vi "DetectDataProcessor.vi"(8 "error in (no error)":errorcluster, 11 "Microscope in":refnum<class "Microscope.lvclass">) -> (0 "error out":errorcluster, 3 "Microscope out":refnum<class "Microscope.lvclass">)   [LabVIEW 2020, in "Microscope.lvlib" / "Microscope.lvclass"]
uses:
  Microscope.lvclass
  Logic Layer/QuickNote/QuickNote/QuickNote.lvclass
  E:/Development/DevHardSoftware/MicroscopyFramework/Model/Logic Layer/DataProcessor/DataProcessor/DataProcessor.lvclass
  Logic Layer/DataLogger/DataLogger/DataLogger.lvclass
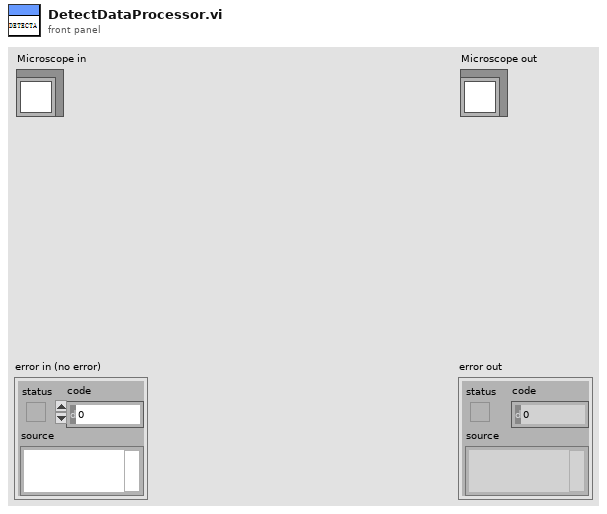
[diagram p1: front panel]
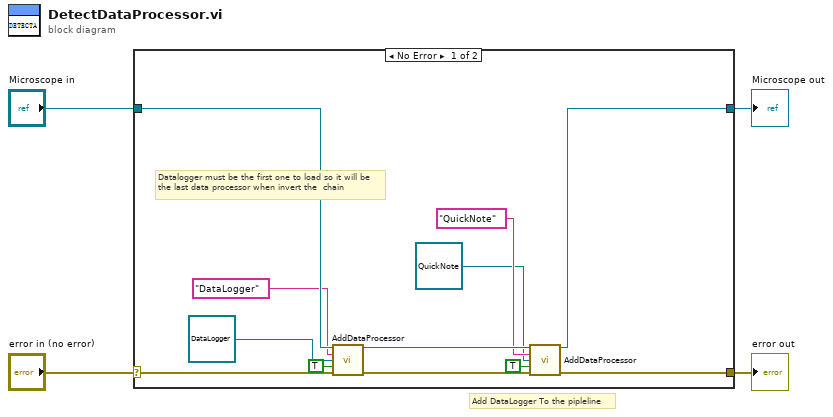
[diagram p0: block diagram]
diagram:
  # "Add DataLogger To the pipleline"
  n1 = case shown="No Error" "error in (no error)" {
    selector: "error in (no error)" -> [w16 w18]
    tunnel: [w9 w18] -> w3
    tunnel: [w11 w17] -> w1
    tunnel: "Microscope in" -> [w14 w17]
    frame No Error {
      # "Datalogger must be the first one to load so it will be\nthe last data processor when invert the  chain"
      n2 = call-dynamic "AddDataProcessor.vi"("Microscope in"=w14, "Label"="DataLogger", "DataProcessor"=refnum<class "DataLogger.lvclass"> refnum ("DataLogger.lvlib:DataLogger.lvclass"), "RegisterInPipleline?(F)"=TRUE, "error in (no error)"=w16) -> ("Microscope out"=w12:refnum<class "Microscope.lvclass">, "error out"=w15:errorcluster)  [unwired: 9 in]
      n3 = call-dynamic "AddDataProcessor.vi"("Microscope in"=w12, "Label"="QuickNote", "DataProcessor"=refnum<class "QuickNote.lvclass"> refnum ("QuickNote.lvlib:QuickNote.lvclass"), "RegisterInPipleline?(F)"=TRUE, "error in (no error)"=w15) -> ("Microscope out"=w11:refnum<class "Microscope.lvclass">, "error out"=w9:errorcluster)  [unwired: 9 in]
    }
    frame Error {
    }
  }
  "error out" <- w3
  "Microscope out" <- w1
